vi "meetCriteria.vi"(8 "error in (no error)":errorcluster, 10 "Persons In":refnum<class "Person.lvclass">[](array[class]), 11 "AndCriteria in":refnum<class "AndCriteria.lvclass">) -> (0 "error out":errorcluster, 2 "Persons Out":refnum<class "Person.lvclass">[](array[class]), 3 "AndCriteria out":refnum<class "AndCriteria.lvclass">)   [LabVIEW 2018, in "AndCriteria.lvclass"]
uses:
  AndCriteria.lvclass
  Person Class/Person.lvclass
  AndCriteria.lvclass/AndCriteria.ctl
  Criteria Class/Criteria.lvclass
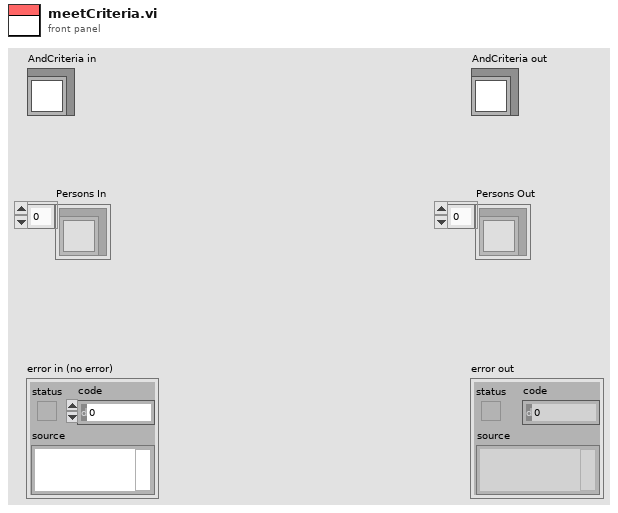
[diagram p1: front panel]
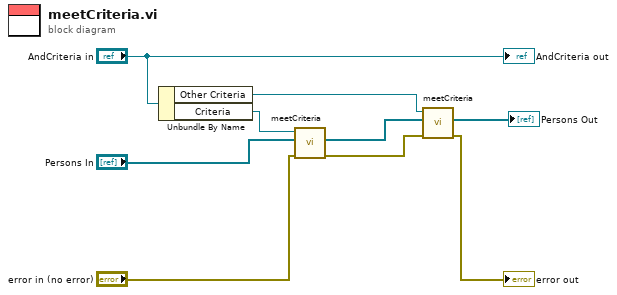
[diagram p0: block diagram]
diagram:
  n1 = Unbundle By Name("AndCriteria in") -> ("Other Criteria"=w5:refnum<class "Criteria.lvclass">, "Criteria"=w8:refnum<class "Criteria.lvclass">)
  n2 = call-dynamic "meetCriteria.vi"("error in (no error)"="error in (no error)", "Persons In"="Persons In", "Criteria in"=w8) -> ("error out"=w2:errorcluster, "Persons Out"=w6:refnum<class "Person.lvclass">[])  [unwired: 6 in, 1 out]
  n3 = call-dynamic "meetCriteria.vi"("error in (no error)"=w2, "Persons In"=w6, "Criteria in"=w5) -> ("error out"=→"error out":errorcluster, "Persons Out"=→"Persons Out":refnum<class "Person.lvclass">[])  [unwired: 6 in, 1 out]
  "AndCriteria out" <- "AndCriteria in"
